vi "DataLoggingSessionError Event Callback.vi"(4 "Error Event":refnum<user-event>, 5 "Event Data":cluster{"sender":refnum<k24>, "e":refnum<k24>}, 6 "Data Logging Manager Ref":T1, 7 "Event Common Data":T2) -> ()   [LabVIEW 2020, in "NI_VS Data Logging API.lvlib"]
uses:
  <vilib>/NI VeriStand/Execution/DataLogging/NI_VS Data Logging API.lvlib
  <vilib>/NI VeriStand/Execution/DataLogging/IDataLogging Ref.ctl
  NationalInstruments.VeriStand.ClientAPI
  <vilib>/NI VeriStand/Execution/DataLogging/Data Logging Session Error Event Data.ctl
  NationalInstruments.VeriStand
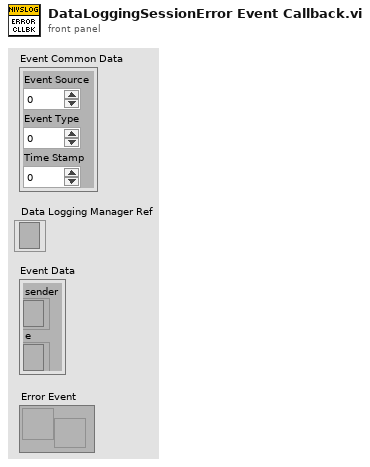
[diagram p1: front panel]
types:
  T1 = typedef "NI_VS Data Logging API.lvlib/IDataLogging Ref.ctl" = refnum<k24>
  T2 = cluster{"Event Source":i32, "Event Type":u32, "Time Stamp":u32}
  T3 = typedef "NI_VS Data Logging API.lvlib/Data Logging Session Error Event Data.ctl" = cluster{"Session Name":string, "Error":errorcluster}
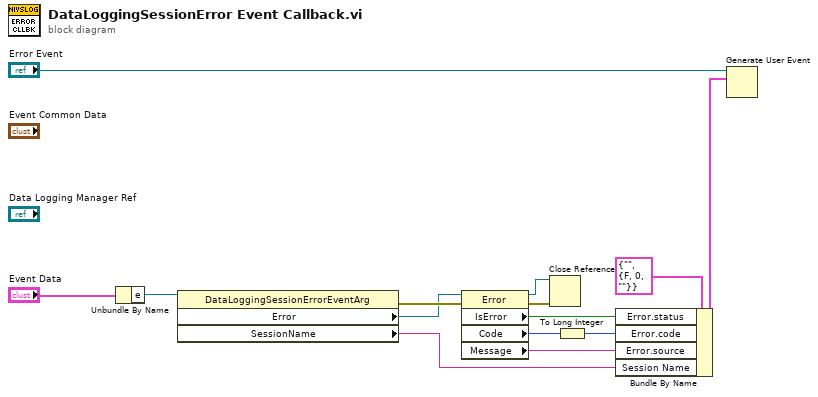
[diagram p0: block diagram]
diagram:
  n1 = Unbundle By Name("Event Data") -> ("e"=w10:refnum<k24>)
  n2 = property class="DataLoggingSessionErrorEventArg"(reference=w10) -> (error out=w4:errorcluster, "Error"=w3:refnum<k24>, "SessionName"=w2:string)  [unwired: 1 in, 1 out]
  n3 = property class="Error"(reference=w3, error in=w4) -> (reference out=w8:refnum<k24>, error out=w5:errorcluster, "IsError"=w6:bool, "Code"=w9:u32, "Message"=w7:string)
  n4 = Close Reference(reference=w8, error in (no error)=w5) -> ()  [unwired: 1 out]
  n5 = To Long Integer(number=w9) -> (32bit integer=w1:i32)
  n6 = Bundle By Name(cluster=T3 {"Session Name"="", "Error"={"status"=FALSE, "code"=0, "source"=""}} ("event data"), "Error.status"=w6, "Error.code"=w1, "Error.source"=w7, "Session Name"=w2) -> (w11:T3)
  n7 = Generate User Event(user event="Error Event", event data cluster=w11) -> ()  [unwired: 2 in, 2 out]
